vi "Remove_Shortcut.vi"(8 "error in (no error)":errorcluster, 10 "shortcut":string, 11 "IB_Source_File in":refnum<class "IB_Source_File.lvclass">) -> (0 "error out":errorcluster, 1 "removed shortcut":refnum<class "IB_Shortcut.lvclass">, 2 "shortcut address":string, 3 "IB_Source_File out":refnum<class "IB_Source_File.lvclass">)   [LabVIEW 2020, in "IB_Source_File.lvclass"]
uses:
  <vilib>/AppBuilder/IB_Classes/Source/File/IB_Source_File.lvclass
  <vilib>/AppBuilder/IB_Classes/Source/File/IB_Source_File.lvclass/IB_Source_File.ctl
  <vilib>/AppBuilder/IB_Classes/Shortcut/IB_Shortcut.lvclass
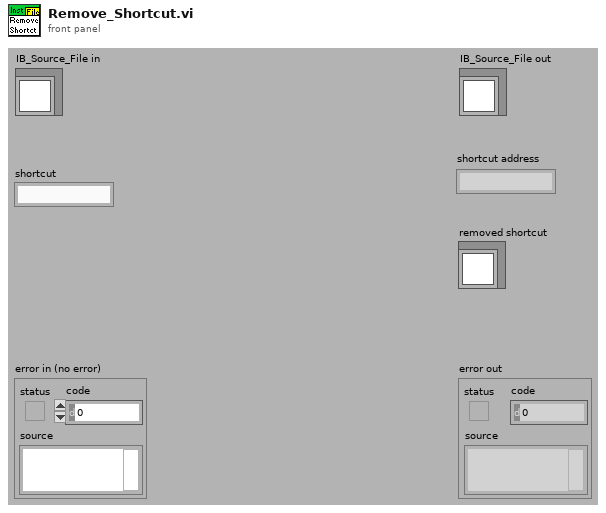
[diagram p1: front panel]
types:
  T1 = typedef "IB_Shortcut.ctl" = cluster{"name":string, "destIndex":i32, "subDir":string, "address":string}
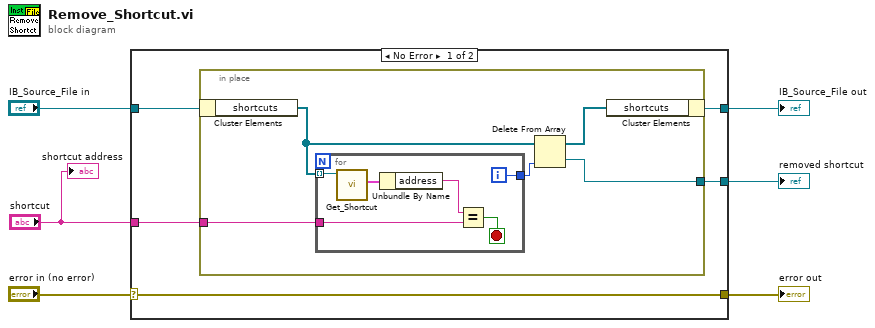
[diagram p0: block diagram]
diagram:
  n1 = case shown="No Error" "error in (no error)" {
    selector: "error in (no error)" -> [w11 w24]
    tunnel: [w11 w24] -> w5
    tunnel: [w7 w23] -> w3
    tunnel: "IB_Source_File in" -> [w8 w23]
    tunnel: "shortcut" -> [w10 _]
    tunnel: [w9 _] -> w2
    frame No Error {
      n2 = in-place {
        in-place-border: w10 -> [w16]
        in-place-border: [w12] -> w9
        n3 = in-place-cluster #1(w8) -> ("shortcuts"=w15:refnum<class "IB_Shortcut.lvclass">[])
        n4 = for {
          tunnel: w15 -> [w22] mode=indexing
          tunnel: w16 -> [w20]
          tunnel: [w18] -> w14
          i -> [w18]
          stop <- w19 stop-if-true
          n5 = call <vilib>:"Get_Shortcut.vi"("Class in"=w22) -> ("data"=w21:T1)  [unwired: 1 in, 9 out]
          n6 = Unbundle By Name(w21) -> ("address"=w17:string)
          n7 = Equal?(x=w17, y=w20) -> (x = y?=w19:bool)
        }
        n8 = Delete From Array(array=w15, index=w14) -> (deleted portion=w12:refnum<class "IB_Shortcut.lvclass">, array with subset deleted=w13:refnum<class "IB_Shortcut.lvclass">[])  [unwired: 1 in]
        n9 = in-place-cluster #1("shortcuts"=w13) -> (w7:refnum<class "IB_Source_File.lvclass">)
      }
    }
    frame Error {
    }
  }
  "error out" <- w5
  "IB_Source_File out" <- w3
  "removed shortcut" <- w2
  "shortcut address" <- "shortcut"
